vi "RTS Door Timer.vi"(8 "Error In":errorcluster, 10 "Time Limit (sec)":dbl, 11 "Reset Timer?":bool) -> (0 "Error Out":errorcluster, 2 "Times Up?":bool, 3 "Elapsed Time (sec)":dbl)   [LabVIEW 2016]
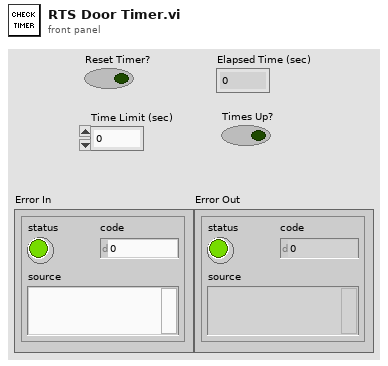
[diagram p1: front panel]
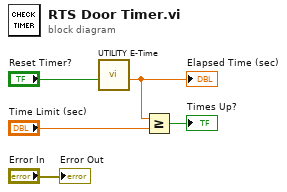
[diagram p0: block diagram]
diagram:
  n1 = call "UTILITY E-Time.vi"("Reset"="Reset Timer?") -> ("Elapsed Time (sec)"=w4:dbl)  [unwired: 8 in, 2 out]
  "Elapsed Time (sec)" <- w4
  n2 = Greater Or Equal?(x=w4, y="Time Limit (sec)") -> (x >= y?=→"Times Up?":bool)
  "Error Out" <- "Error In"
